vi "Open.vi"(8 "error in":errorcluster, 11 "Services Token":string) -> (0 "error out":errorcluster, 3 "Web App Handle":T1)   [LabVIEW 2013, in "Web Messaging API.lvlib"]
doc: "Initializes the Web Messaging Connection. The Services token is available at https://myRIO.niwsc.com"
uses:
  Web Messaging API.lvlib
  Web Messaging Handle.ctl
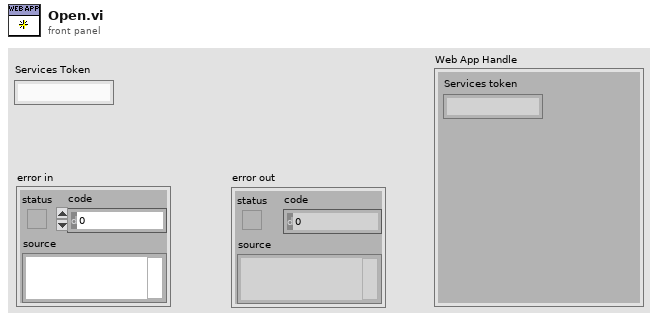
[diagram p1: front panel]
types:
  T1 = typedef "Web Messaging API.lvlib/Web Messaging Handle.ctl" = cluster{"Services token":string}
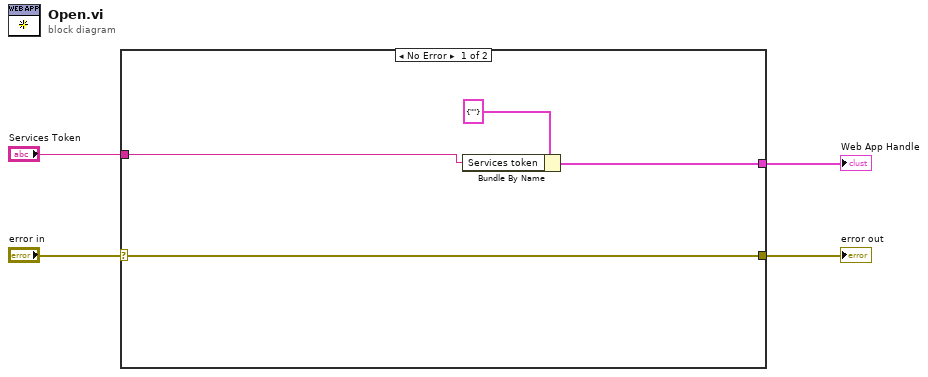
[diagram p0: block diagram]
diagram:
  n1 = case shown="No Error" "error in" {
    selector: "error in" -> [w6 w9]
    tunnel: [w6 w9] -> w3
    tunnel: [w8 _] -> w1
    tunnel: "Services Token" -> [w7 _]
    frame No Error {
      n2 = Bundle By Name(cluster=T1 {"Services token"=""} ("Web App Handle 1"), "Services token"=w7) -> (w8:T1)
    }
    frame Error {
    }
  }
  "error out" <- w3
  "Web App Handle" <- w1
